vi "Esercitazione 4 - For Loop.vi"() -> ()   [LabVIEW 2018]
panel:
  out "Numeric":i32
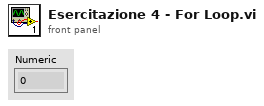
[diagram p1: front panel]
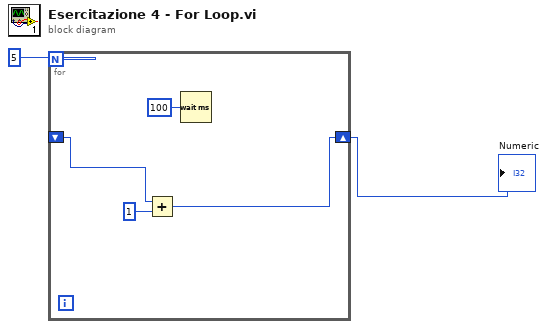
[diagram p0: block diagram]
diagram:
  n1 = for {
    N: 5 -> [_]
    shift-right: [w4] -> w1
    shift-left: _ -> [w3]
    n2 = Add(x=w3, y=1) -> (x+y=w4:i32)
    n3 = Wait (ms)(milliseconds to wait=u32 100) -> ()  [unwired: 1 out]
  }
  "Numeric" <- w1
